vi "Analog Input - Synchronization.vi"() -> ()   [LabVIEW 2022 SP3]
doc: "This example demonstrates how to acquire a continuous amount of data (Waveform) using the DAQ device's internal clock. It also shows how to synchronize two devices for different device families (E Series, S Series, M Series, X Series, DSA, and SC Express), to simultaneously acquire the data.\n\nFor instructions on how to connect your signals to the DAQ device, refer to your device documentation."
uses:
  <vilib>/Utility/error.llb/DialogType.ctl
  <vilib>/DAQmx/read.llb/DAQmx Read (Analog 1D Wfm NChan NSamp).vi
  <vilib>/DAQmx/create/channels.llb/DAQmx Create Channel (AI-Voltage-Basic).vi
  <vilib>/DAQmx/configure/timing.llb/DAQmx Timing (Sample Clock).vi
  <vilib>/DAQmx/configure/trigger.llb/DAQmx Start Trigger (Digital Edge).vi
  <vilib>/DAQmx/miscellaneous.llb/DAQmx Fill In Error Info.vi
  <resource>/objmgr/daqmx.rc
panel:
  in  "Synchronization Type*":T1(ring)
  in  "Stop":bool
  out "Waveform Graph":waveform(dbl)[](graph)
  in  "Samples per Loop":i32=100
  in  "Sample Rate":dbl=1000.0
  in  "Slave Physical Channel(s)":tag="Dev1/ai0"
  in  "Master Physical Channel(s)":tag="Dev1/ai0"
  # "Channel Settings"
  # "Acquired Data"
  # "Timing Settings"
  # "*Note:  This example is intended to show low level synchronization of various devices.\nDSA, S Series, X Series, and SC Express devices support including channels from multiple devices in a single task.\nDAQmx automatically synchronizes the devices in such a task.  See the DAQmx Help>>\nDevice Considerations>>Multi Device Tasks section for further details."
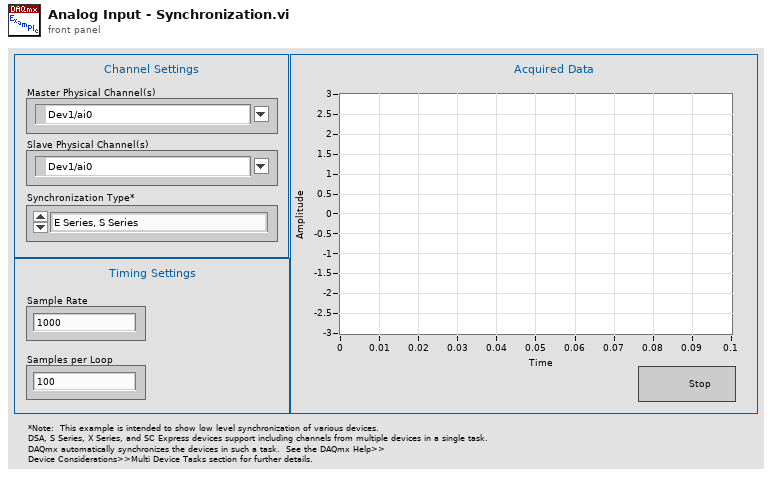
[diagram p1: front panel]
types:
  T1 = enum16{"E Series, S Series", "M Series (PCI)", "M Series (PXI)", "DSA Sample Clock Timebase", "DSA Reference Clock", "X Series (PCIe)", "X Series (PXIe), SC Express"}
  T2 = typedef "DialogType.ctl" = u16
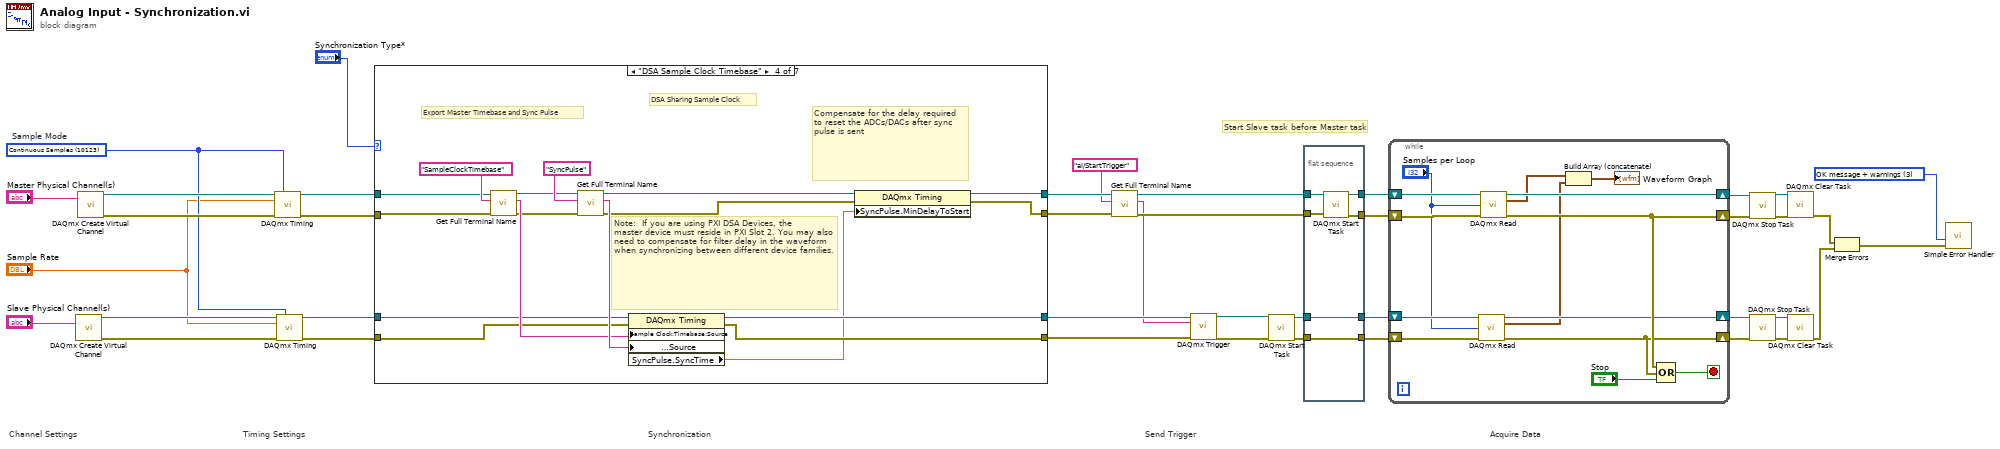
[diagram p0: block diagram]
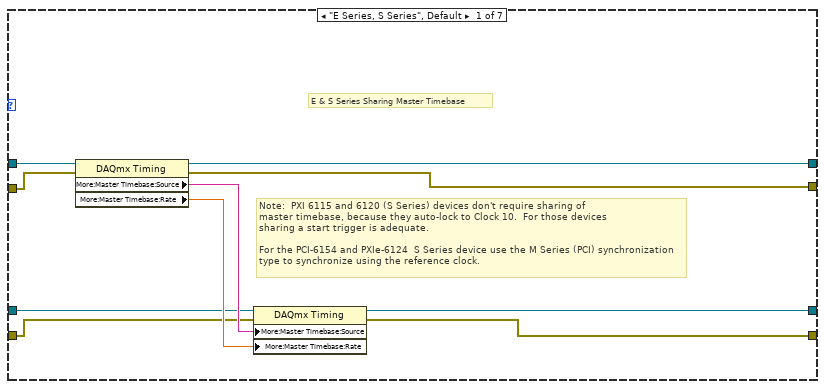
[diagram p2: hidden frame]
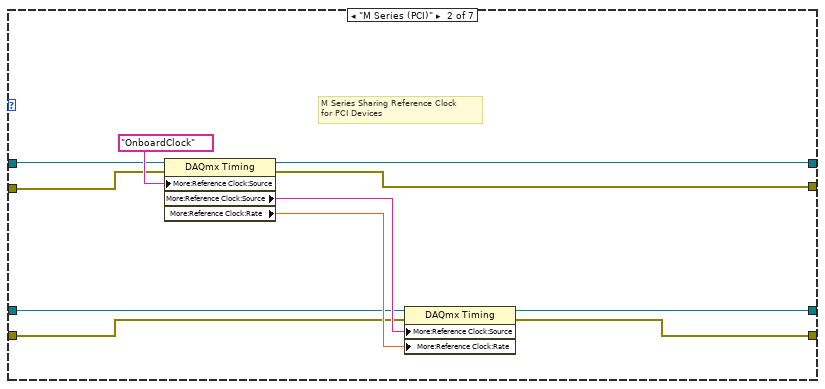
[diagram p3: hidden frame]
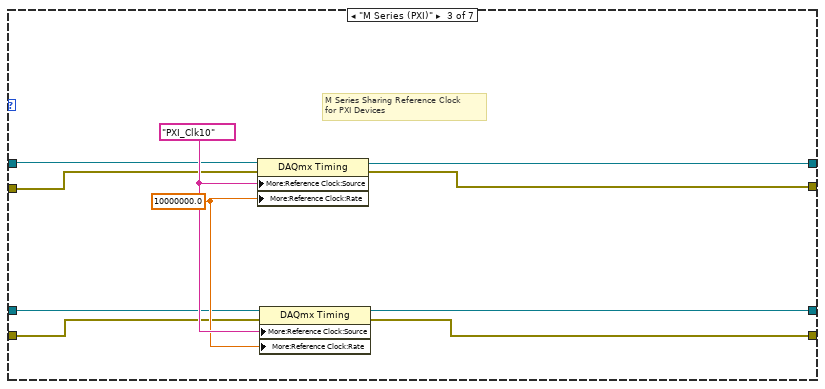
[diagram p4: hidden frame]
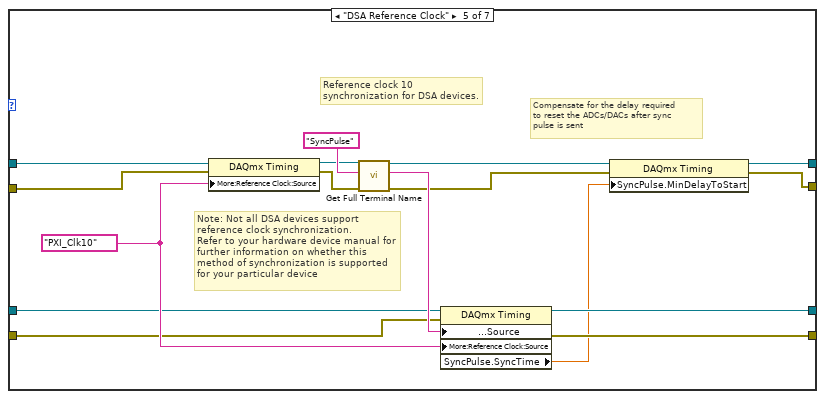
[diagram p5: hidden frame]
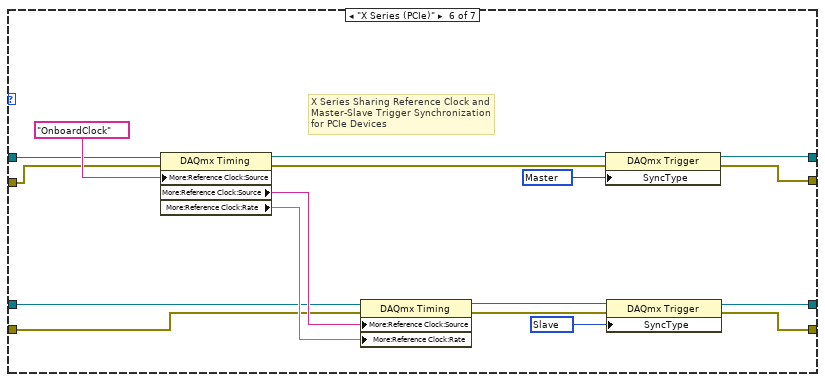
[diagram p6: hidden frame]
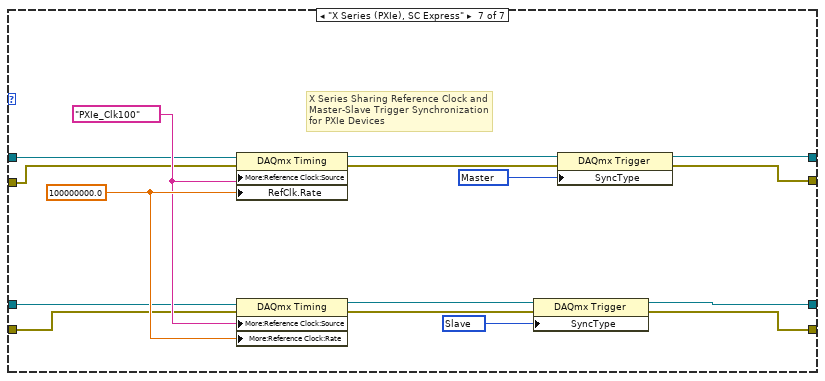
[diagram p7: hidden frame]
diagram:
  w1 = T2 3 items=["no dialog", "OK message", "continue or stop message", "OK message + warnings", "continue/stop + warnings"] ("type of dialog (OK msg:1)")
  w13 = 10123 items=["Finite Samples"=10178, "Continuous Samples"=10123, "Hardware Timed Single Point"=12522]  # Sample Mode
  # "Send Trigger"
  # "Acquire Data"
  # "Synchronization"
  # "Timing Settings"
  # "Channel Settings"
  # "Start Slave task before Master task"
  n1 = call-poly <vilib>:"DAQmx Create Virtual Channel.vi"("physical channels"="Slave Physical Channel(s)") -> ("task out"=w15:refnum<k21>, "error out"=w17:errorcluster)  [unwired: 13 in]
  n2 = call-poly <vilib>:"DAQmx Create Virtual Channel.vi"("physical channels"="Master Physical Channel(s)") -> ("task out"=w21:refnum<k21>, "error out"=w20:errorcluster)  [unwired: 13 in]
  n3 = call-poly <vilib>:"DAQmx Timing.vi"("task/channels in"=w21, "sample mode"=w13, "rate"="Sample Rate", "error in"=w20) -> ("task out"=w18:refnum<k21>, "error out"=w19:errorcluster)  [unwired: 10 in]
  n4 = call-poly <vilib>:"DAQmx Timing.vi"("task/channels in"=w15, "sample mode"=w13, "rate"="Sample Rate", "error in"=w17) -> ("task out"=w16:refnum<k21>, "error out"=w14:errorcluster)  [unwired: 10 in]
  n5 = case shown="\"DSA Sample Clock Timebase\"" "Synchronization Type*" {
    tunnel: [w51 w58 w70 w83 w102 w117 w131] -> w11
    tunnel: [w50 w57 w69 w82 w101 w116 w130] -> w8
    tunnel: [w49 w59 w71 w77 w94 w112 w132] -> w7
    tunnel: [w46 w56 w67 w76 w93 w113 w129] -> w6
    tunnel: w19 -> [w45 w55 w66 w81 w97 w109 w125]
    tunnel: w18 -> [w44 w54 w65 w80 w98 w108 w126]
    tunnel: w16 -> [w43 w53 w64 w79 w96 w107 w124]
    tunnel: w14 -> [w42 w52 w63 w78 w95 w106 w123]
    frame "E Series, S Series", Default {
      # "Note:  PXI 6115 and 6120 (S Series) devices don't require sharing of\nmaster timebase, because they auto-lock to Clock 10.  For those devices\nsharing a start trigger is adequate.\n\nFor the PCI-6154 and PXIe-6124  S Series device use the M Series (PCI) synchronization \ntype to synchronize using the reference clock."
      # "E & S Series Sharing Master Timebase"
      n6 = property class="DAQmx Timing"(reference=w44, error in=w45) -> (reference out=w49:refnum<k21>, error out=w46:errorcluster, "More:Master Timebase:Source"=w48:tag, "More:Master Timebase:Rate"=w47:dbl)
      n7 = property class="DAQmx Timing"(reference=w43, error in=w42, "More:Master Timebase:Source"=w48, "More:Master Timebase:Rate"=w47) -> (reference out=w51:refnum<k21>, error out=w50:errorcluster)
    }
    frame "M Series (PCI)" {
      # "M Series Sharing Reference Clock\nfor PCI Devices"
      n8 = property class="DAQmx Timing"(reference=w54, error in=w55, "More:Reference Clock:Source"=tag "OnboardClock" ("RefClk.Src")) -> (reference out=w59:refnum<k21>, error out=w56:errorcluster, "More:Reference Clock:Source"=w61:tag, "More:Reference Clock:Rate"=w60:dbl)
      n9 = property class="DAQmx Timing"(reference=w53, error in=w52, "More:Reference Clock:Source"=w61, "More:Reference Clock:Rate"=w60) -> (reference out=w58:refnum<k21>, error out=w57:errorcluster)
    }
    frame "M Series (PXI)" {
      w68 = 10000000.0 ("RefClk.Rate")
      w72 = tag "PXI_Clk10" ("RefClk.Src")
      # "M Series Sharing Reference Clock\nfor PXI Devices"
      n10 = property class="DAQmx Timing"(reference=w65, error in=w66, "More:Reference Clock:Source"=w72, "More:Reference Clock:Rate"=w68) -> (reference out=w71:refnum<k21>, error out=w67:errorcluster)
      n11 = property class="DAQmx Timing"(reference=w64, error in=w63, "More:Reference Clock:Source"=w72, "More:Reference Clock:Rate"=w68) -> (reference out=w70:refnum<k21>, error out=w69:errorcluster)
    }
    frame "DSA Sample Clock Timebase" {
      # "Compensate for the delay required\nto reset the ADCs/DACs after sync\npulse is sent"
      # "Export Master Timebase and Sync Pulse"
      # "Note:  If you are using PXI DSA Devices, the \nmaster device must reside in PXI Slot 2. You may also need to compensate for filter delay in the waveform when synchronizing between different device families."
      # "DSA Sharing Sample Clock"
      n12 = call "Get Full Terminal Name.vi"("error in"=w81, "Local Terminal Name"="SampleClockTimebase", "task/channels in"=w80) -> ("error out"=w87:errorcluster, "Terminal Name with Device Prefix"=w88:tag, "task out"=w85:refnum<k21>)  [unwired: 6 in]
      n13 = call "Get Full Terminal Name.vi"("error in"=w87, "Local Terminal Name"="SyncPulse", "task/channels in"=w85) -> ("error out"=w74:errorcluster, "Terminal Name with Device Prefix"=w89:tag, "task out"=w75:refnum<k21>)  [unwired: 6 in]
      n14 = property class="DAQmx Timing"(reference=w79, error in=w78, "Sample Clock:Timebase:Source"=w88, "More:Synchronization Pulse:Source"=w89) -> (reference out=w83:refnum<k21>, error out=w82:errorcluster, "SyncPulse.SyncTime"=w73:dbl)
      n15 = property class="DAQmx Timing"(reference=w75, error in=w74, "SyncPulse.MinDelayToStart"=w73) -> (reference out=w77:refnum<k21>, error out=w76:errorcluster)
    }
    frame "DSA Reference Clock" {
      w100 = tag "PXI_Clk10" ("RefClk.Src")
      # "Compensate for the delay required\nto reset the ADCs/DACs after sync\npulse is sent"
      # "Note: Not all DSA devices support\nreference clock synchronization.\nRefer to your hardware device manual for\nfurther information on whether this \nmethod of synchronization is supported\nfor your particular device"
      # "Reference clock 10\nsynchronization for DSA devices."
      n16 = property class="DAQmx Timing"(reference=w98, error in=w97, "More:Reference Clock:Source"=w100) -> (reference out=w104:refnum<k21>, error out=w103:errorcluster)
      n17 = call "Get Full Terminal Name.vi"("error in"=w103, "Local Terminal Name"="SyncPulse", "task/channels in"=w104) -> ("error out"=w91:errorcluster, "Terminal Name with Device Prefix"=w99:tag, "task out"=w92:refnum<k21>)  [unwired: 6 in]
      n18 = property class="DAQmx Timing"(reference=w96, error in=w95, "More:Synchronization Pulse:Source"=w99, "More:Reference Clock:Source"=w100) -> (reference out=w102:refnum<k21>, error out=w101:errorcluster, "SyncPulse.SyncTime"=w90:dbl)
      n19 = property class="DAQmx Timing"(reference=w92, error in=w91, "SyncPulse.MinDelayToStart"=w90) -> (reference out=w94:refnum<k21>, error out=w93:errorcluster)
    }
    frame "X Series (PCIe)" {
      w110 = 15889 items=["None"=10230, "Master"=15888, "Slave"=15889] ("SyncType")
      w111 = 15888 items=["None"=10230, "Master"=15888, "Slave"=15889] ("SyncType")
      # "X Series Sharing Reference Clock and \nMaster-Slave Trigger Synchronization \nfor PCIe Devices"
      n20 = property class="DAQmx Timing"(reference=w108, error in=w109, "More:Reference Clock:Source"=tag "OnboardClock" ("RefClk.Src")) -> (reference out=w115:refnum<k21>, error out=w114:errorcluster, "More:Reference Clock:Source"=w122:tag, "More:Reference Clock:Rate"=w121:dbl)
      n21 = property class="DAQmx Timing"(reference=w107, error in=w106, "More:Reference Clock:Source"=w122, "More:Reference Clock:Rate"=w121) -> (reference out=w119:refnum<k21>, error out=w118:errorcluster)
      n22 = property class="DAQmx Trigger"(reference=w115, error in=w114, "SyncType"=w111) -> (reference out=w112:refnum<k21>, error out=w113:errorcluster)
      n23 = property class="DAQmx Trigger"(reference=w119, error in=w118, "SyncType"=w110) -> (reference out=w117:refnum<k21>, error out=w116:errorcluster)
    }
    frame "X Series (PXIe), SC Express" {
      w128 = 100000000.0 ("RefClk.Rate")
      w138 = 15889 items=["None"=10230, "Master"=15888, "Slave"=15889] ("SyncType")
      w137 = 15888 items=["None"=10230, "Master"=15888, "Slave"=15889] ("SyncType")
      w127 = tag "PXIe_Clk100" ("RefClk.Src")
      # "X Series Sharing Reference Clock and \nMaster-Slave Trigger Synchronization \nfor PXIe Devices"
      n24 = property class="DAQmx Timing"(reference=w126, error in=w125, "More:Reference Clock:Source"=w127, "RefClk.Rate"=w128) -> (reference out=w135:refnum<k21>, error out=w136:errorcluster)
      n25 = property class="DAQmx Timing"(reference=w124, error in=w123, "More:Reference Clock:Source"=w127, "More:Reference Clock:Rate"=w128) -> (reference out=w133:refnum<k21>, error out=w134:errorcluster)
      n26 = property class="DAQmx Trigger"(reference=w133, error in=w134, "SyncType"=w138) -> (reference out=w131:refnum<k21>, error out=w130:errorcluster)
      n27 = property class="DAQmx Trigger"(reference=w135, error in=w136, "SyncType"=w137) -> (reference out=w132:refnum<k21>, error out=w129:errorcluster)
    }
  }
  n28 = call "Get Full Terminal Name.vi"("error in"=w6, "Local Terminal Name"="ai/StartTrigger", "task/channels in"=w7) -> ("error out"=w4:errorcluster, "Terminal Name with Device Prefix"=w2:tag, "task out"=w5:refnum<k21>)  [unwired: 6 in]
  n29 = call-poly <vilib>:"DAQmx Trigger.vi"("task/channels in"=w11, "source"=w2, "error in"=w8) -> ("task out"=w10:refnum<k21>, "error out"=w9:errorcluster)  [unwired: 11 in]
  n30 = call <vilib>:"DAQmx Start Task.vi"("task/channels in"=w10, "error in"=w9) -> ("task out"=w41:refnum<k21>, "error out"=w40:errorcluster)  [unwired: 12 in]
  n31 = flat-sequence {
    tunnel: w41 -> [w144]
    tunnel: w40 -> [w143]
    tunnel: [w144] -> w37
    tunnel: [w143] -> w36
    tunnel: [w142] -> w38
    tunnel: [w141] -> w39
    tunnel: w5 -> [w140]
    tunnel: w4 -> [w139]
    frame #0 {
      n32 = call <vilib>:"DAQmx Start Task.vi"("task/channels in"=w140, "error in"=w139) -> ("task out"=w141:refnum<k21>, "error out"=w142:errorcluster)  [unwired: 12 in]
    }
  }
  n33 = while {
    shift-right: [w154] -> w34
    shift-left: w38 -> [w155]
    shift-right: [w151] -> w30
    shift-left: w36 -> [w152]
    shift-right: [w157] -> w35
    shift-left: w39 -> [w156]
    shift-right: [w150] -> w31
    shift-left: w37 -> [w153]
    stop <- w158 stop-if-true
    n34 = call-poly <vilib>:"DAQmx Read.vi"("task/channels in"=w153, "number of samples per channel"="Samples per Loop", "error in"=w152) -> ("task out"=w150:refnum<k21>, "data"=w145:waveform(dbl)[], "error out"=w151:errorcluster)  [unwired: 10 in]
    n35 = call-poly <vilib>:"DAQmx Read.vi"("task/channels in"=w156, "number of samples per channel"="Samples per Loop", "error in"=w155) -> ("task out"=w157:refnum<k21>, "data"=w146:waveform(dbl)[], "error out"=w154:errorcluster)  [unwired: 10 in]
    n36 = Build Array (concatenate)(w146, w145) -> (→"Waveform Graph":waveform(dbl)[])
    n37 = Compound Arithmetic op=OR(w154, w151, "Stop") -> (w158:bool)
  }
  n38 = call <vilib>:"DAQmx Stop Task.vi"("task/channels in"=w35, "error in"=w34) -> ("task out"=w32:refnum<k21>, "error out"=w33:errorcluster)  [unwired: 12 in]
  n39 = call <vilib>:"DAQmx Stop Task.vi"("task/channels in"=w31, "error in"=w30) -> ("task out"=w28:refnum<k21>, "error out"=w29:errorcluster)  [unwired: 12 in]
  n40 = call <vilib>:"DAQmx Clear Task.vi"("task in"=w32, "error in"=w33) -> ("error out"=w27:errorcluster)  [unwired: 13 in]
  n41 = call <vilib>:"DAQmx Clear Task.vi"("task in"=w28, "error in"=w29) -> ("error out"=w26:errorcluster)  [unwired: 13 in]
  n42 = Merge Errors(w27, w26) -> (w25:errorcluster)
  n43 = call <vilib>:"Simple Error Handler.vi"("type of dialog (OK msg:1)"=w1, "error in (no error)"=w25) -> ()  [unwired: 3 in, 5 out]
